vi "PH_Beamline_Chief.Data to Settings.vi"(1 "data":i8[](array[numeric])) -> (0 "Settings":T1)   [LabVIEW 2014, in "PH_Beamline_Chief.lvlib"]
uses:
  PH_Beamline_Chief.lvlib
  PH_Beamline_Chief.Settings.ctl
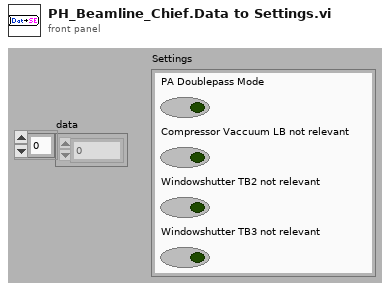
[diagram p1: front panel]
types:
  T1 = typedef "PH_Beamline_Chief.lvlib/PH_Beamline_Chief.Settings.ctl" = cluster{"PA Doublepass Mode":bool, "Compressor Vaccuum LB not relevant":bool, "Windowshutter TB2 not relevant":bool, "Windowshutter TB3 not relevant":bool}
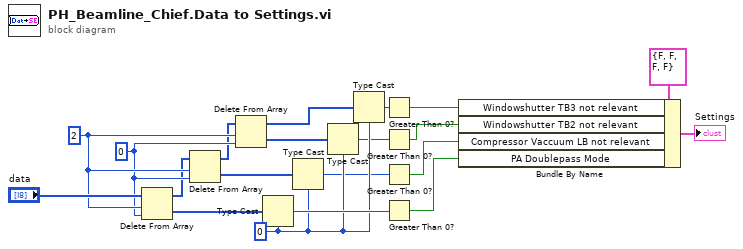
[diagram p0: block diagram]
diagram:
  w13 = i16 0
  w16 = 2 ("length")
  w15 = 0 ("index")
  n1 = Delete From Array(array="data", length=w16, index=w15) -> (deleted portion=w8:i8[], array with subset deleted=w9:i8[])
  n2 = Delete From Array(array=w9, length=w16, index=w15) -> (deleted portion=w6:i8[], array with subset deleted=w7:i8[])
  n3 = Delete From Array(array=w7, length=w16, index=w15) -> (deleted portion=w5:i8[], array with subset deleted=w4:i8[])
  n4 = Type Cast(type=w13, x=w8) -> (*(type *) &x=w14:i16)
  n5 = Type Cast(type=w13, x=w6) -> (*(type *) &x=w12:i16)
  n6 = Type Cast(type=w13, x=w5) -> (*(type *) &x=w11:i16)
  n7 = Type Cast(type=w13, x=w4) -> (*(type *) &x=w10:i16)
  n8 = Greater Than 0?(x=w10) -> (x > 0?=w3:bool)
  n9 = Greater Than 0?(x=w11) -> (x > 0?=w2:bool)
  n10 = Greater Than 0?(x=w12) -> (x > 0?=w1:bool)
  n11 = Greater Than 0?(x=w14) -> (x > 0?=w17:bool)
  n12 = Bundle By Name(cluster=T1 {"PA Doublepass Mode"=FALSE, "Compressor Vaccuum LB not relevant"=FALSE, "Windowshutter TB2 not relevant"=FALSE, "Windowshutter TB3 not relevant"=FALSE} ("Settings"), "Windowshutter TB3 not relevant"=w3, "Windowshutter TB2 not relevant"=w2, "Compressor Vaccuum LB not relevant"=w1, "PA Doublepass Mode"=w17) -> (→"Settings":T1)
